vi "Verify Required Options.vi"(0 "Required Options":string, 5 "Reported Options":string, 11 "error in (no error)":errorcluster) -> (4 "Mismatch? (True = Mismatch)":bool, 15 "error out":errorcluster)   [LabVIEW 2018]
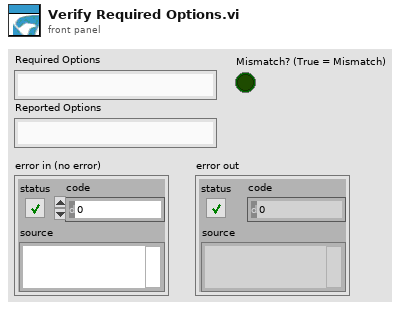
[diagram p1: front panel]
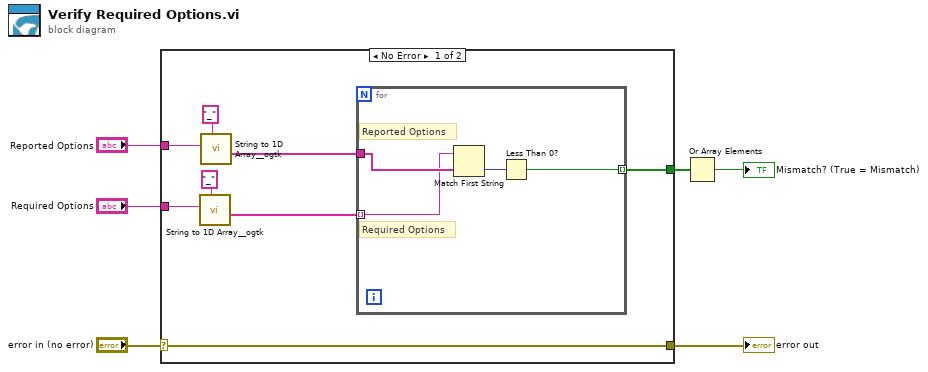
[diagram p0: block diagram]
diagram:
  n1 = case shown="No Error" "error in (no error)" {
    selector: "error in (no error)" -> [w10 w19]
    tunnel: [w10 w19] -> w5
    tunnel: "Reported Options" -> [w14 _]
    tunnel: "Required Options" -> [w11 _]
    tunnel: [w7 _] -> w2
    frame No Error {
      n2 = call <userlib>:"String to 1D Array__ogtk.vi"("delimiter (Tab)"="_", "string"=w11) -> ("Array of Strings"=w8:string[])  [unwired: 9 in]
      n3 = call <userlib>:"String to 1D Array__ogtk.vi"("delimiter (Tab)"="_", "string"=w14) -> ("Array of Strings"=w9:string[])  [unwired: 9 in]
      n4 = for {
        tunnel: w9 -> [w16]
        tunnel: w8 -> [w15] mode=indexing
        tunnel: [w17] -> w7 mode=indexing
        # "Reported Options"
        # "Required Options"
        n5 = Match First String(2:w16, 3:w15) -> (0:w18:i32)  [unwired: 1 out]
        n6 = Less Than 0?(x=w18) -> (x < 0?=w17:bool)
      }
    }
    frame Error {
    }
  }
  "error out" <- w5
  n7 = Or Array Elements(Boolean array=w2) -> (logical OR=→"Mismatch? (True = Mismatch)":bool)
